vi "HTTP GET.vi"(8 "error in (no error)":errorcluster, 10 "Endpoint":string, 11 "REST_Client in":refnum<class "REST_Client.lvclass">) -> (0 "error out":errorcluster, 1 "body":string, 2 "headers":string, 3 "REST_Client out":refnum<class "REST_Client.lvclass">)   [LabVIEW 2020, in "REST_Client.lvclass"]
uses:
  REST_Client.lvclass
  <vilib>/httpClient/LabVIEWHTTPClient.lvlib
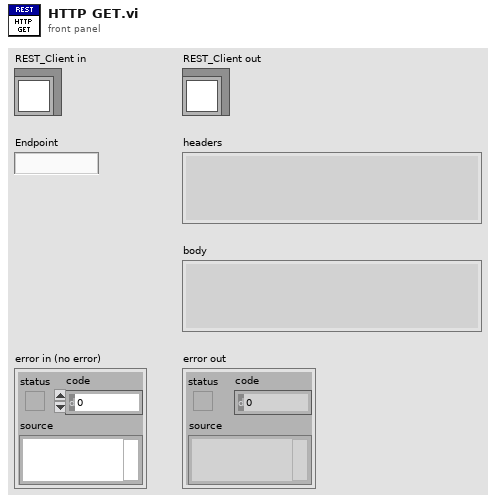
[diagram p1: front panel]
types:
  T1 = typedef "LabVIEWHTTPClient.lvlib/ClientHandle.ctl" = refnum<k1>
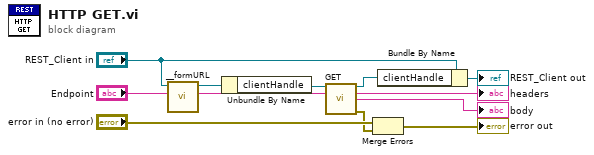
[diagram p0: block diagram]
diagram:
  n1 = call "__formURL.vi"("endPoint"="Endpoint", "REST_Client in"="REST_Client in") -> ("URL"=w4:string, "REST_Client out"=w2:refnum<class "REST_Client.lvclass">)  [unwired: 8 in]
  n2 = Unbundle By Name(w2) -> ("clientHandle"=w1:T1)
  n3 = call <vilib>:"GET.vi"("client handle"=w1, "url"=w4) -> ("client handle out"=w10:T1, "headers"=→"headers":string, "body"=→"body":string, "error out"=w7:errorcluster)  [unwired: 10 in]
  n4 = Merge Errors("error in (no error)", w7) -> (→"error out":errorcluster)
  n5 = Bundle By Name(cluster="REST_Client in", "clientHandle"=w10) -> (→"REST_Client out":refnum<class "REST_Client.lvclass">)
